vi "Read Subordinate Object Queue.vi"(8 "error in (no error)":errorcluster, 9 "Name":string, 11 "Measure Object in":refnum<class "Measure Object.lvclass">) -> (0 "error out":errorcluster, 1 "Object Enqueuer":refnum<class "Message Enqueuer.lvclass">, 2 "Found?":bool, 3 "Measure Object out":refnum<class "Measure Object.lvclass">)   [LabVIEW 2015, in "Measure Object.lvclass"]
uses:
  Measure Object.lvclass
  <vilib>/ActorFramework/Message Enqueuer/Message Enqueuer.lvclass
  Measure Object.lvclass/Measure Object.ctl
  <vilib>/ActorFramework/Actor/Actor.lvclass/Actor.ctl
  <vilib>/ActorFramework/Message Enqueuer/Message Enqueuer.lvclass/Message Enqueuer.ctl
  Read Name.vi
  <vilib>/ActorFramework/Message Enqueuer/Init from Existing Queue.vi
  <vilib>/ActorFramework/Actor/Actor.lvclass
panel:
  in  "Self Enqueuer":refnum<class "Message Enqueuer.lvclass">
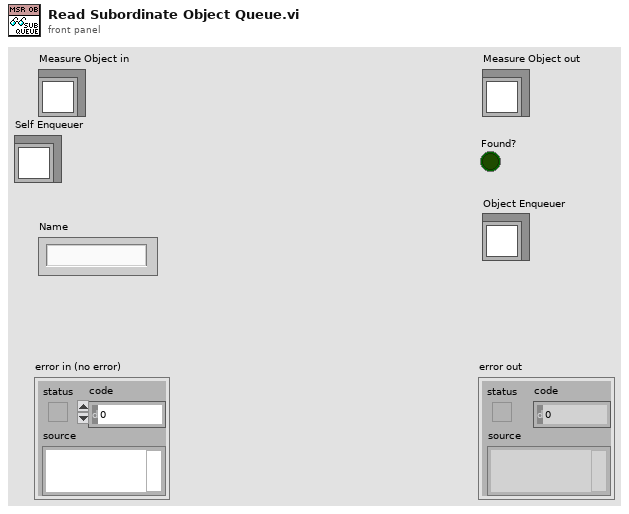
[diagram p1: front panel]
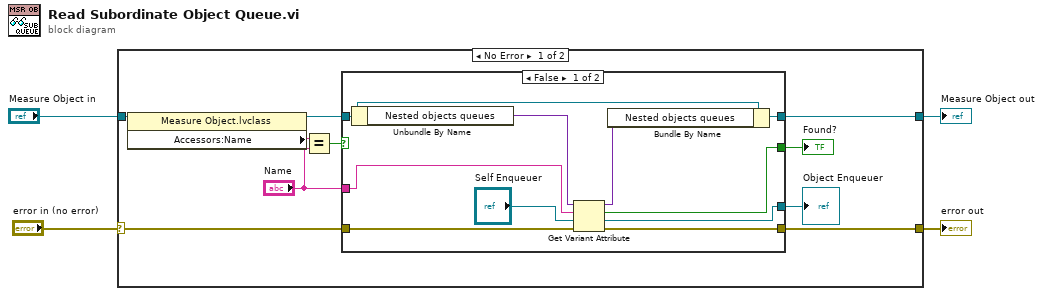
[diagram p0: block diagram]
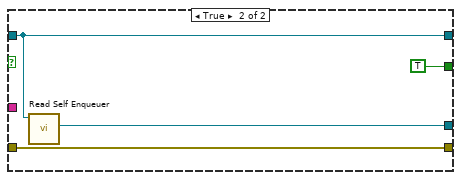
[diagram p2: hidden frame]
diagram:
  n1 = case shown="No Error" "error in (no error)" {
    selector: "error in (no error)" -> [w14 w30]
    tunnel: [w12 w30] -> w3
    tunnel: [w13 w29] -> w1
    tunnel: "Measure Object in" -> [w11 w29]
    frame No Error {
      n2 = property class="Measure Object.lvclass"(reference=w11) -> (reference out=w10:refnum<class "Measure Object.lvclass">, "Accessors:Name"=w9:string)  [unwired: 1 in, 1 out]
      n3 = Equal?(x=w9, y="Name") -> (x = y?=w5:bool)
      n4 = case shown="False" w5 {
        tunnel: w14 -> [w23 w25]
        tunnel: [w22 w26] -> w13
        tunnel: [w20 w25] -> w12
        tunnel: w10 -> [w19 w26]
        tunnel: "Name" -> [w18 _]
        tunnel: [w16 TRUE] -> w7
        tunnel: [w15 w28] -> w6
        frame False {
          n5 = Unbundle By Name(w19) -> ("Nested objects queues"=w24:variant)
          n6 = Get Variant Attribute(Variant=w24, name=w18, default value (empty Variant)="Self Enqueuer", error in=w23) -> (duplicate Variant=w21:variant, found=w16:bool, value=w15:refnum<class "Message Enqueuer.lvclass">, error out=w20:errorcluster)
          n7 = Bundle By Name(cluster=w19, "Nested objects queues"=w21) -> (w22:refnum<class "Measure Object.lvclass">)
        }
        frame True {
          n8 = call <vilib>:"Read Self Enqueuer.vi"("Actor"=w26) -> ("Self Enqueuer"=w28:refnum<class "Message Enqueuer.lvclass">)  [unwired: 10 in]
        }
      }
      "Found?" <- w7
      "Object Enqueuer" <- w6
    }
    frame Error {
    }
  }
  "error out" <- w3
  "Measure Object out" <- w1
